vi "setDescription.vi"(8 "error in (no error)":errorcluster, 10 "description":string="Unknown", 11 "HouseBlend in":refnum<class "HouseBlend.lvclass">) -> (0 "error out":errorcluster, 3 "HouseBlend out":refnum<class "HouseBlend.lvclass">)   [LabVIEW 2018, in "HouseBlend.lvclass"]
uses:
  HouseBlend.lvclass
  Beverage Class/Beverage.lvclass
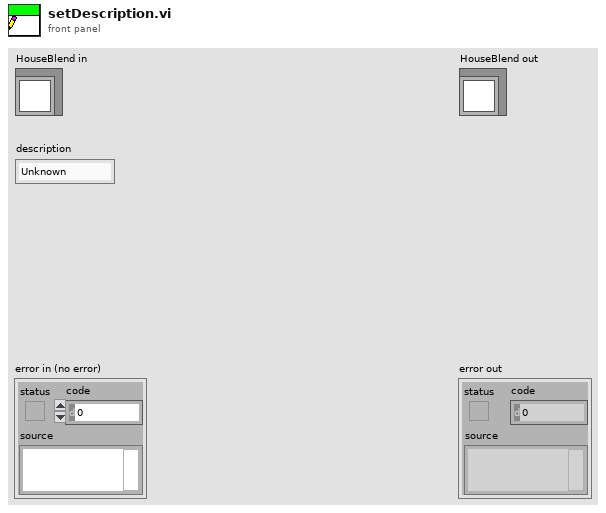
[diagram p1: front panel]
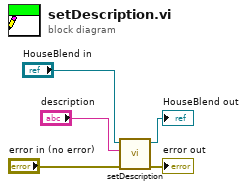
[diagram p0: block diagram]
diagram:
  n1 = call-parent "setDescription.vi"("error in (no error)"="error in (no error)", "description"="description", "Beverage in"="HouseBlend in") -> ("error out"=→"error out":errorcluster, "Beverage out"=→"HouseBlend out":refnum<class "HouseBlend.lvclass">)  [unwired: 7 in]
